vi "DL-Create IPC.vi"() -> (8 "IPC":T1)   [LabVIEW 2020]
uses:
  Typedefs/DL-IPC.ctl
  Typedefs/DL-Configuration.ctl
  Typedefs/DL-Channel Spec.ctl
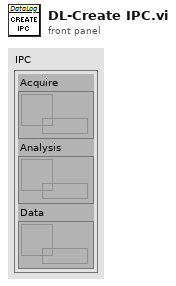
[diagram p1: front panel]
types:
  T1 = typedef "DL-IPC.ctl" = cluster{"Acquire":refnum<queue>, "Analysis":refnum<queue>, "Data":refnum<queue>}
  T2 = typedef "DL-Configuration.ctl" = cluster{"Folder":path, "Filestem":string, "Device":string, "Fs (Hz)":dbl, "T (s)":dbl, "AI":T3[], "frame size (s)":dbl, ".wav file":bool, "Trigger":enum16{"Internal", "External"}}
  T3 = typedef "DL-Channel Spec.ctl" = cluster{"active":bool, "name":string}
  T4 = cluster{"queue out":refnum<queue>, "queue out":refnum<queue>, "queue out":refnum<queue>}
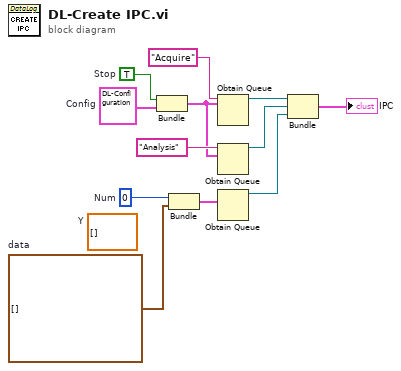
[diagram p0: block diagram]
diagram:
  w1 = waveform(dbl)[] []  # data
  w2 = TRUE  # Stop
  w9 = 0  # Num
  (unwired) dbl[][] []  # Y
  w4 = T2 {"Folder"=path "", "Filestem"="", "Device"="", "Fs (Hz)"=0.0, "T (s)"=0.0, "AI"=[], "frame size (s)"=0.0, ".wav file"=FALSE, "Trigger"=enum."Internal"}  # Config
  n1 = Bundle("Stop"=w2, "Config"=w4) -> (w3:cluster{"Stop":bool, "Config":T2})  [unwired: 1 in]
  n2 = Bundle("Num"=w9, "data"=w1) -> (w11:cluster{"Num":i32, "data":waveform(dbl)[]})  [unwired: 1 in]
  n3 = Obtain Queue(name (unnamed)="Acquire", element data type=w3) -> (queue out=w12:refnum<queue>)  [unwired: 3 in, 2 out]
  n4 = Obtain Queue(name (unnamed)="Analysis", element data type=w3) -> (queue out=w6:refnum<queue>)  [unwired: 3 in, 2 out]
  n5 = Obtain Queue(element data type=w11) -> (queue out=w10:refnum<queue>)  [unwired: 4 in, 2 out]
  n6 = Bundle("queue out"=w12, "queue out"=w6, "queue out"=w10) -> (→"IPC":T4)  [unwired: 1 in]
